vi "Parse Used Session and Name.vi"(2 "name":string, 3 "Section Name(\"\" as Default)":string) -> (0 "used name":string)   [LabVIEW 2017, in "INI-Static-Variable-Support.lvlib"]
uses:
  INI-Static-Variable-Support.lvlib
  <userlib>/_NEVSTOP/Communicable State Machine(CSM)/Communicable State Machine.lvlib
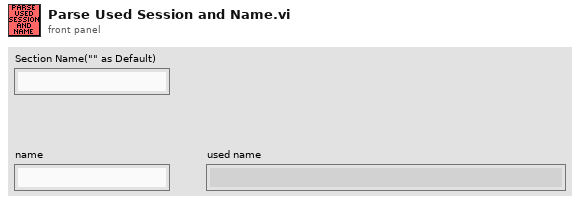
[diagram p1: front panel]
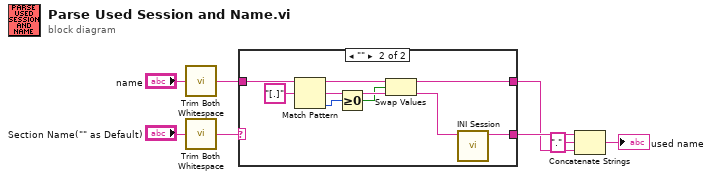
[diagram p0: block diagram]
diagram:
  n1 = call <userlib>:"Trim Both Whitespace.vi"("String"="name") -> ("Trimmed String"=w1:string)  [unwired: 1 in]
  n2 = call <userlib>:"Trim Both Whitespace.vi"("String"="Section Name(\"\" as Default)") -> ("Trimmed String"=w2:string)  [unwired: 1 in]
  n3 = case shown="\"\"" w2 {
    selector: w2 -> [w9 _]
    tunnel: w1 -> [w10 w19]
    tunnel: [w10 w11] -> w4
    tunnel: [w9 w16] -> w6
    frame Default {
    }
    frame "" {
      n4 = Match Pattern(string=w19, regular expression="[.]") -> (before substring=w15:string, after substring=w14:string, offset past match=w17:i32)  [unwired: 1 in, 1 out]
      n5 = Greater Or Equal To 0?(x=w17) -> (x >= 0?=w13:bool)
      n6 = Swap Values(12:w15, 13:w13, 14:w14) -> (1:w11:string, 3:w12:string)
      n7 = call "INI Session.vi"("Section Name(\"\" as Default)"=w12) -> ("App.Name"=w16:string)  [unwired: 10 in]
    }
  }
  n8 = Concatenate Strings(w6, "." ("string"), w4) -> (→"used name":string)
